vi "Read DMA.vi"(8 "error in (no error)":errorcluster, 9 "Timed out?":bool, 10 "Injection Event Data Cluster in":T1 {"Shot Info Array"."Results"."Off-Stage Avg Current" format="%#.6g"; "Shot Info Array"."Results"."Total Voltage Pulses" format="%#.6g"; "Shot Info Array"."Results"."Off-Stage Min Current" format="%#.6g"; "Shot Info Array"."Results"."Off-Stage Max Current" format="%#.6g"}, 11 "DMA Ref":refnum<k20>) -> (0 "error out":errorcluster, 1 "Data":fxp<+/-,32,8>[](array[numeric]), 2 "Injection Event Data Cluster":T1 {"Shot Info Array"."Results"."Off-Stage Avg Current" format="%#.6g"; "Shot Info Array"."Results"."Total Voltage Pulses" format="%#.6g"; "Shot Info Array"."Results"."Off-Stage Min Current" format="%#.6g"; "Shot Info Array"."Results"."Off-Stage Max Current" format="%#.6g"}, 3 "DMA Ref":refnum<k20>)   [LabVIEW 2015, in "Fuel Injection Addon Engine.lvlib"]
uses:
  Fuel Injection Addon Engine.lvlib
  Types/Injector Event Data Cluster.ctl
  RT Analysis/Controls/Shot Information Control.ctl
  Types/Boost Stage Current Measurements Cluster Control.ctl
  <vilib>/Utility/error.llb/Error Cluster From Error Code.vi
  <vilib>/rvi/errors/niLvFpgaAdjustHostInterfaceError.vi
  <vilib>/rvi/interface/nirviMethod/nirviMethod.xnode
  <vilib>/FPGAPlugInAG/Dynamic/niLvFpga_ReadFifo_Dynamic.vi
  <vilib>/rvi/errors/niLvFpgaMergeErrorWithErrorCode.vi
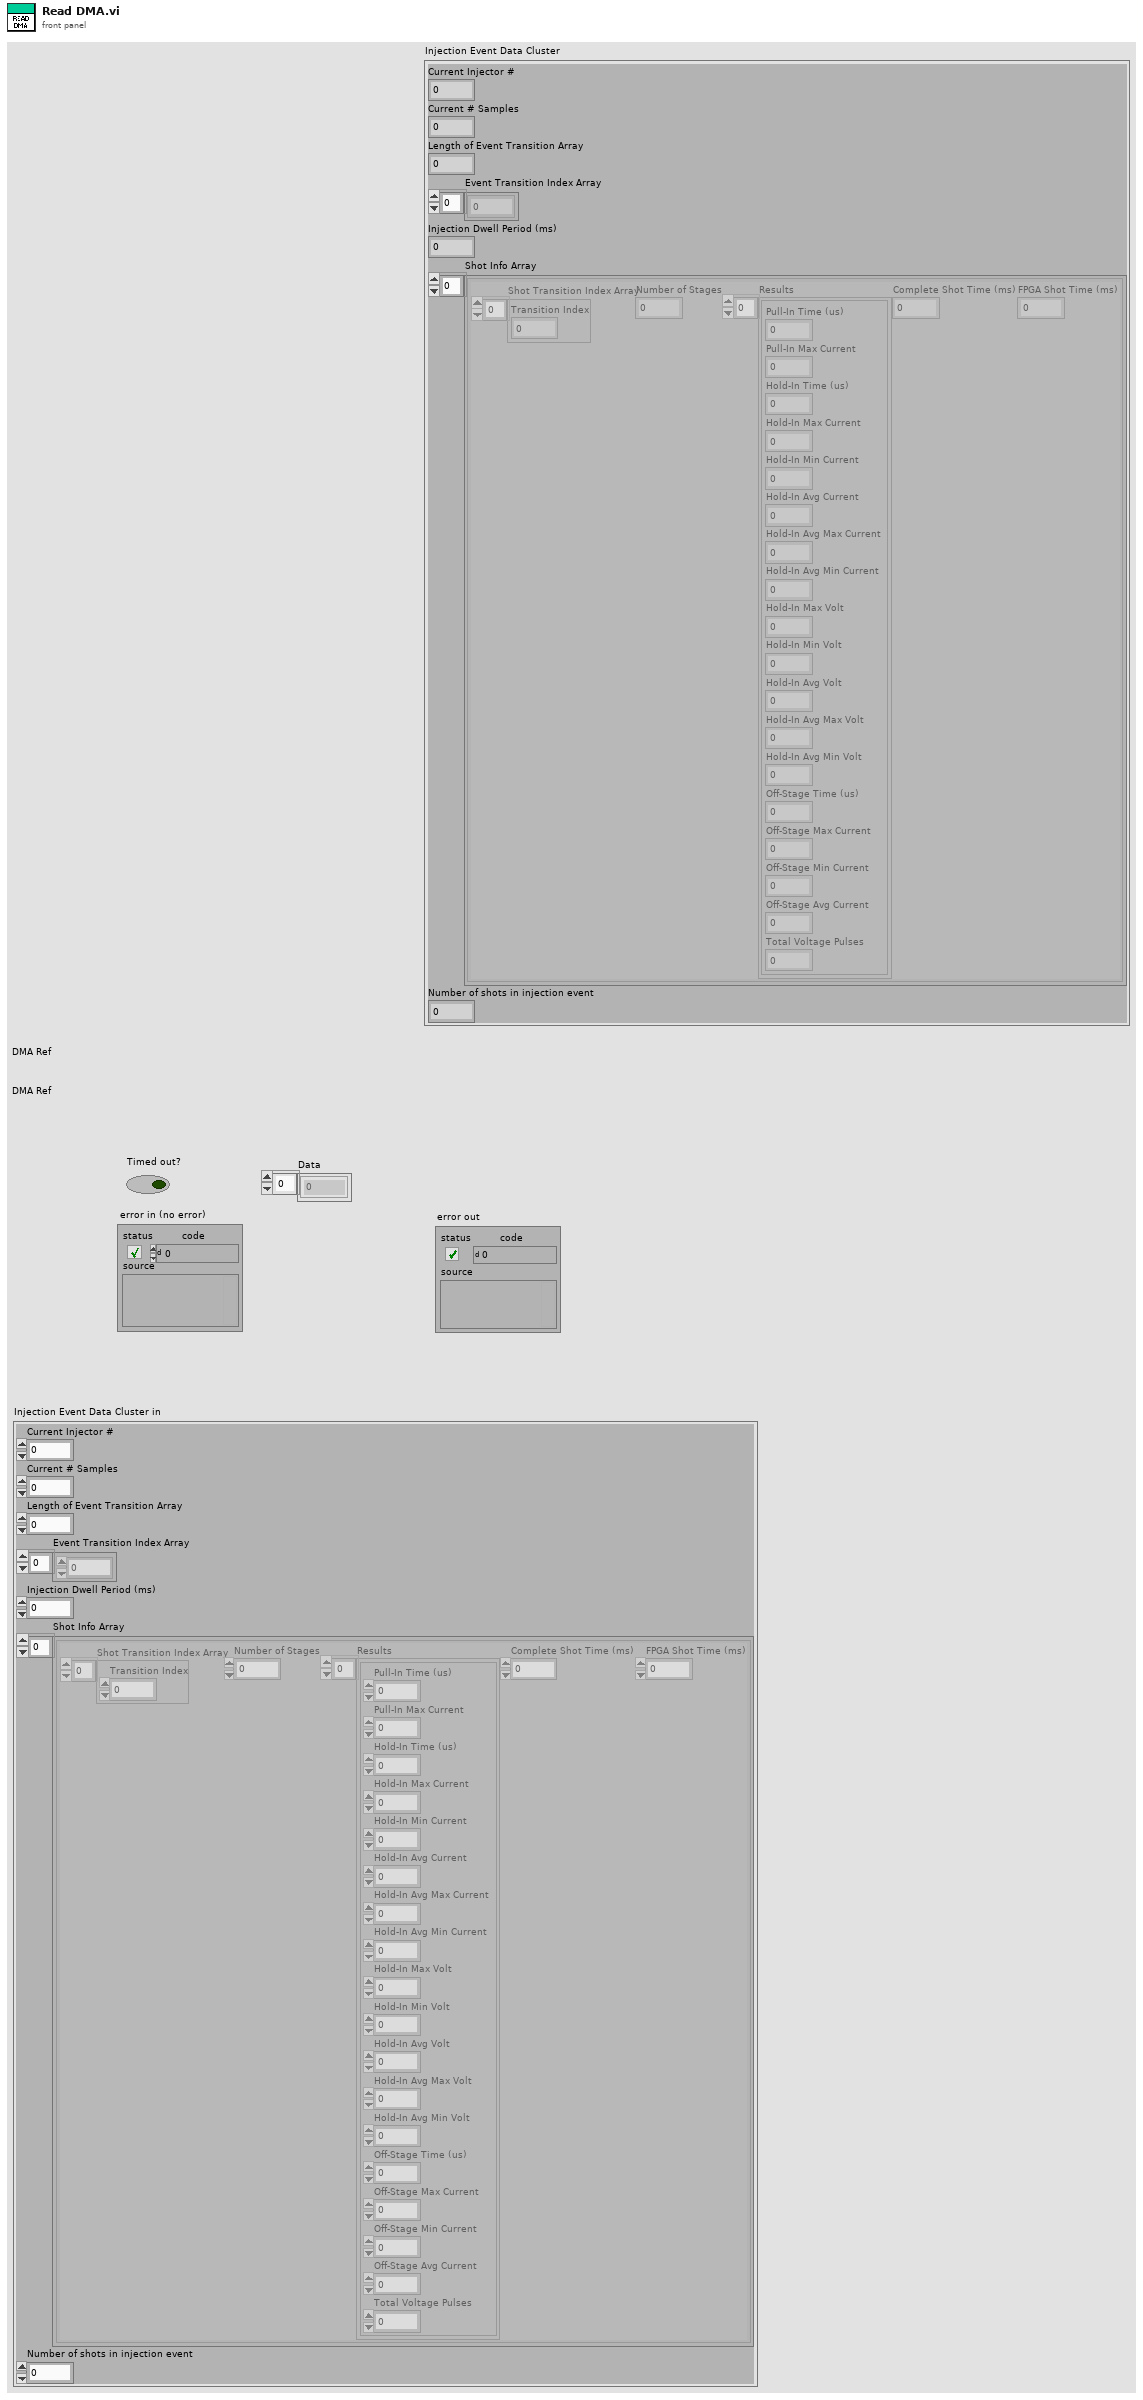
[diagram p1: front panel]
types:
  T1 = typedef "Fuel Injection Addon Engine.lvlib/Injector Event Data Cluster.ctl" = cluster{"Current Injector #":i16, "Current # Samples":i32, "Length of Event Transition Array":i16, "Event Transition Index Array":i32[], "Injection Dwell Period (ms)":dbl, "Shot Info Array":T2[], "Number of shots in injection event":i32}
  T2 = typedef "Fuel Injection Addon Engine.lvlib/Shot Information Control.ctl" = cluster{"Shot Transition Index Array":i32[], "Number of Stages":u16, "Results":T3[], "Complete Shot Time (ms) ":dbl, "FPGA Shot Time (ms)":dbl}
  T3 = typedef "Fuel Injection Addon Engine.lvlib/Boost Stage Current Measurements Cluster Control.ctl" = cluster{"Pull-In Time (us)":dbl, "Pull-In Max Current":dbl, "Hold-In Time (us)":dbl, "Hold-In Max Current":dbl, "Hold-In Min Current":dbl, "Hold-In Avg Current":dbl, "Hold-In Avg Max Current":dbl, "Hold-In Avg Min Current":dbl, "Hold-In Max Volt":dbl, "Hold-In Min Volt":dbl, "Hold-In Avg Volt":dbl, "Hold-In Avg Max Volt":dbl, "Hold-In Avg Min Volt":dbl, "Off-Stage Time (us)":dbl, "Off-Stage Max Current":dbl, "Off-Stage Min Current":dbl, "Off-Stage Avg Current":dbl, "Total Voltage Pulses":dbl}
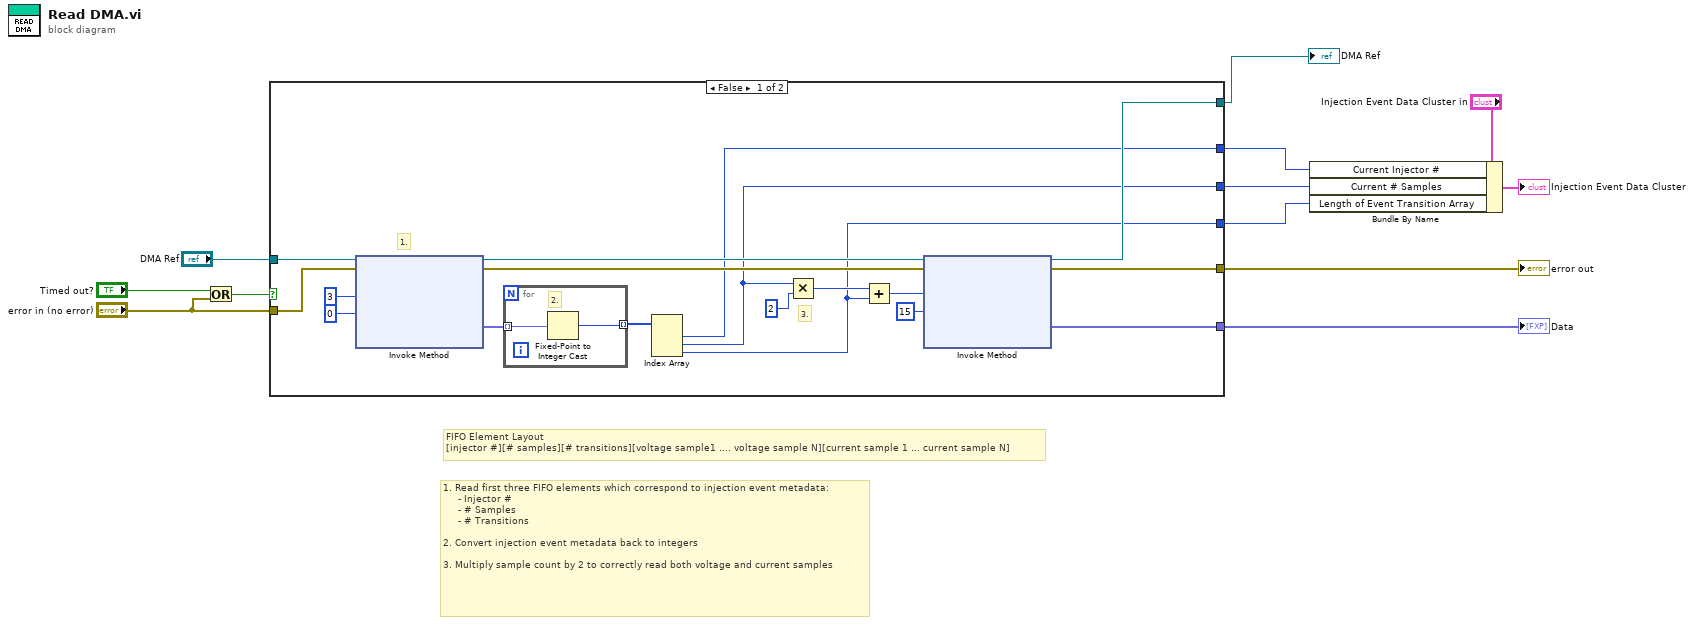
[diagram p0: block diagram]
diagram:
  # "1. Read first three FIFO elements which correspond to injection event metadata: \n     - Injector #\n     - # Samples\n     - # Transitions\n\n2. Convert injection event metadata back to integers\n\n3. Multiply sample count by 2 to correctly read both voltage and current samples"
  # "FIFO Element Layout\n[injector #][# samples][# transitions][voltage sample1 .... voltage sample N][current sample 1 ... current sample N]"
  n1 = Or(x="Timed out?", y="error in (no error)") -> (x .or. y?=w12:bool)
  n2 = case shown="False" w12 {
    tunnel: "error in (no error)" -> [w29 w34]
    tunnel: "DMA Ref" -> [w30 w33]
    tunnel: [w14 w34] -> w9
    tunnel: [w17 w33] -> w1
    tunnel: [w18 _] -> w8
    tunnel: [w15 _] -> w6
    tunnel: [w16 _] -> w3
    tunnel: [w13 _] -> w5
    frame False {
      # "3."
      # "1."
      n3 = xnode "Invoke Method"("FPGA VI Reference In"=w30, "error in"=w29, "Number of Elements"=u32 3, "Timeout (ms)"=0) -> ("FPGA VI Reference Out"=w24:refnum<k20>, "error out"=w23:errorcluster, "Data"=w26:fxp<+/-,32,8>[])  [unwired: 1 out]
      n4 = for {
        tunnel: w26 -> [w32] mode=indexing
        tunnel: [w31] -> w25 mode=indexing
        # "2."
        n5 = Fixed-Point to Integer Cast(1:w32) -> (0:w31:i32)
      }
      n6 = Index Array(array=w25) -> (element #1=w16:i32, element #2=w15:i32, element #3=w13:i32)  [unwired: 3 in]
      n7 = Multiply(x=w15, y=2 ("Timeout (ms)")) -> (x*y=w21:i32)
      n8 = Add(x=w21, y=w13) -> (x+y=w19:i32)
      n9 = xnode "Invoke Method"("FPGA VI Reference In"=w24, "error in"=w23, "Number of Elements"=w19, "Timeout (ms)"=15) -> ("FPGA VI Reference Out"=w17:refnum<k20>, "error out"=w14:errorcluster, "Data"=w18:fxp<+/-,32,8>[])  [unwired: 1 out]
    }
    frame True {
    }
  }
  "error out" <- w9
  "Data" <- w8
  "DMA Ref" <- w1
  n10 = Bundle By Name(cluster="Injection Event Data Cluster in", "Current Injector #"=w3, "Current # Samples"=w6, "Length of Event Transition Array"=w5) -> (→"Injection Event Data Cluster":T1)
